vi "DAC Init Results.vi"(8 "error in":errorcluster, 9 "Log Details?":bool, 10 "tdms file":refnum<k34>, 11 "DAC Heater Ctrl in":refnum<class "DAC Heater Ctrl.lvclass">) -> (0 "error out":errorcluster, 2 "tdms file out":refnum<k34>)   [LabVIEW 2019, in "DAC.lvlib" / "DAC Heater Ctrl.lvclass"]
uses:
  DAC Heater Ctrl.lvclass
  C:/Users/wg/Documents/LV_Projects/test-stand/App/DAC/DAC.lvclass
  DAC.lvclass/DAC.ctl
  DAC Heater Ctrl.lvclass/DAC Heater Ctrl.ctl
  DAC.lvclass
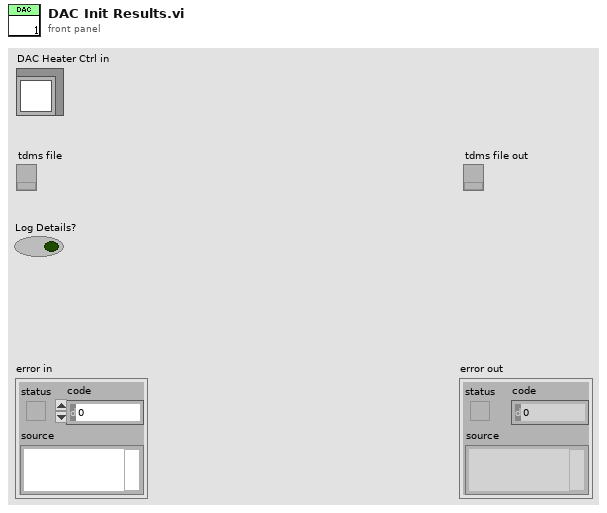
[diagram p1: front panel]
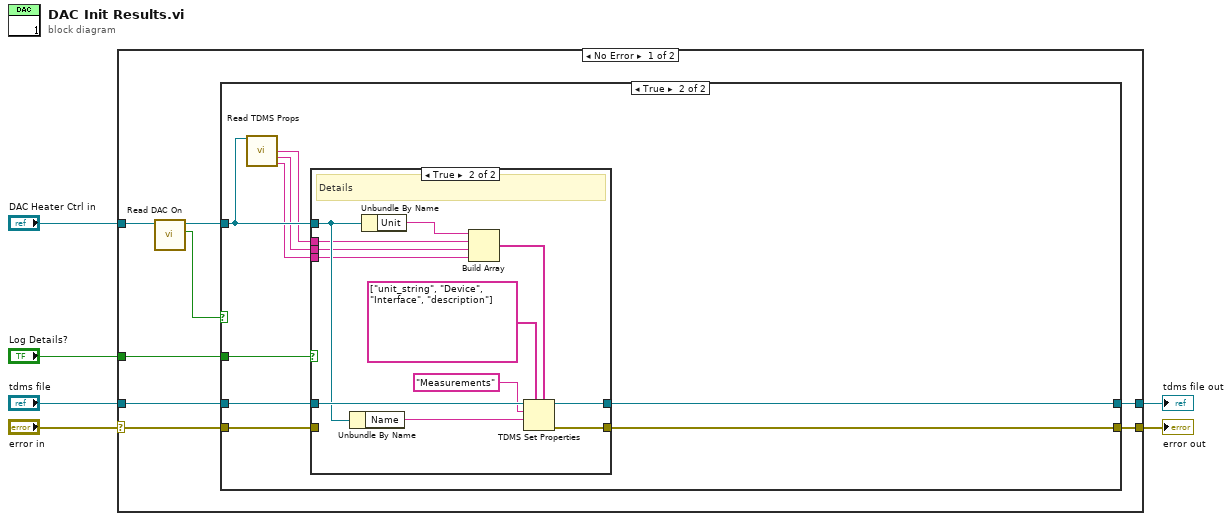
[diagram p0: block diagram]
diagram:
  n1 = case shown="No Error" "error in" {
    selector: "error in" -> [w10 w41]
    tunnel: [w7 w41] -> w6
    tunnel: "DAC Heater Ctrl in" -> [w14 _]
    tunnel: "tdms file" -> [w11 w40]
    tunnel: [w8 w40] -> w5
    tunnel: "Log Details?" -> [w9 _]
    frame No Error {
      n2 = call "Read DAC On.vi"("DAC in"=w14) -> ("DAC On"=w12:bool, "DAC out"=w13:refnum<class "DAC Heater Ctrl.lvclass">)  [unwired: 8 in, 1 out]
      n3 = case shown="True" w12 {
        tunnel: w11 -> [w15 w20]
        tunnel: [w15 w18] -> w8
        tunnel: [w16 w17] -> w7
        tunnel: w13 -> [_ w24]
        tunnel: w10 -> [w16 w25]
        tunnel: w9 -> [_ w19]
        frame False {
        }
        frame True {
          n4 = call "Read TDMS Props.vi"("DAC in"=w24) -> ("DAC Device"=w21:string, "DAC IO"=w22:string, "DAC Description"=w23:string)  [unwired: 10 in, 2 out]
          n5 = case shown="True" w19 {
            tunnel: w20 -> [w27 w39]
            tunnel: [w27 w35] -> w18
            tunnel: [w26 w34] -> w17
            tunnel: w24 -> [_ w32]
            tunnel: w25 -> [w26 _]
            tunnel: w21 -> [_ w30]
            tunnel: w22 -> [_ w29]
            tunnel: w23 -> [_ w28]
            frame False {
            }
            frame True {
              # "Details"
              n6 = Unbundle By Name(w32) -> ("Name"=w33:string)
              n7 = Unbundle By Name(w32) -> ("Unit"=w37:string)
              n8 = Build Array(w37, w30, w29, w28) -> (w36:string[])
              n9 = TDMS Set Properties(5:w36, 7:string[] ["unit_string", "Device", "Interface", "description"] ("property names"), 9:w33, 10:"Measurements" ("group name in (Untitled)"), 11:w39) -> (0:w34:errorcluster, 3:w35:refnum<k34>)  [unwired: 1 in, 2 out]
            }
          }
        }
      }
    }
    frame Error {
    }
  }
  "error out" <- w6
  "tdms file out" <- w5
